vi "PQescapeStringConn.vi"(0 "conn":u64, 5 "to":string, 7 "from":string, 9 "error":i64, 11 "length":u64, 12 "error in (no error)":errorcluster) -> (4 "conn_out":u64, 6 "size_t":u64, 8 "pq_error_out":i64, 15 "error out":errorcluster)   [LabVIEW 2019, in "libpqlv64.lvlib"]
uses:
  libpqlv64.lvlib
  libpq.dll
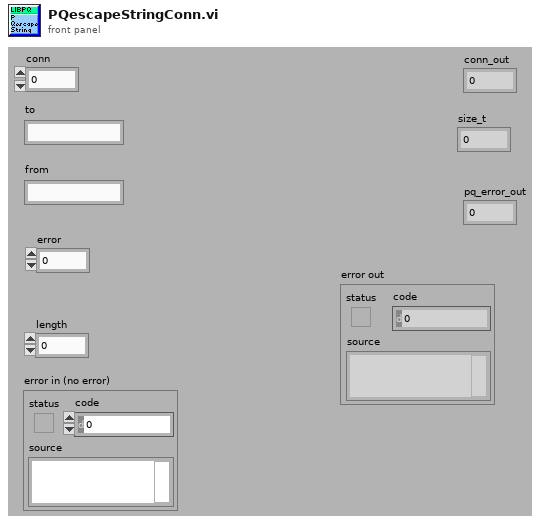
[diagram p1: front panel]
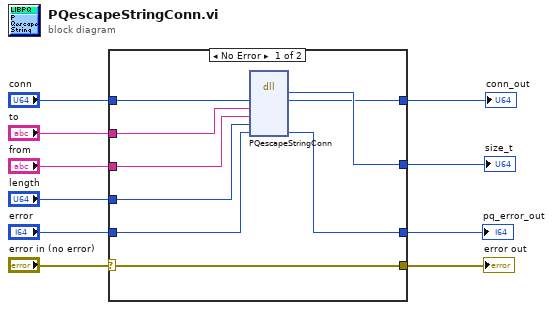
[diagram p0: block diagram]
diagram:
  n1 = case shown="No Error" "error in (no error)" {
    selector: "error in (no error)" -> [w19 w22]
    tunnel: [w19 w22] -> w9
    tunnel: [w18 _] -> w8
    tunnel: [w17 w21] -> w3
    tunnel: "to" -> [w16 _]
    tunnel: "from" -> [w15 _]
    tunnel: "length" -> [w14 _]
    tunnel: "error" -> [w13 w20]
    tunnel: "conn" -> [w12 w21]
    tunnel: [w11 w20] -> w1
    frame No Error {
      n2 = dll-call lib="libpq.*" fn="PQescapeStringConn"("conn"=w12, "to"=w16, "from"=w15, "length"=w14, "error"=w13) -> ("size_t"=w18:u64, "conn"=w17:u64, "error"=w11:i64)  [unwired: 6 in, 2 out]
    }
    frame Error {
    }
  }
  "size_t" <- w8
  "error out" <- w9
  "conn_out" <- w3
  "pq_error_out" <- w1
